vi "NPC3SG Read Data.vi"(0 "VISA resource name in":refnum<visa-resource-name>, 3 "error in":errorcluster) -> (7 "error ende":errorcluster caption="error out" {"code" format="%x"})   [LabVIEW 2010]
uses:
  drivers/Newport NPC3SG/SubNPC3SG.llb/device variables.vi
panel:
  out "Read OK":bool caption="Daten empfangen?"
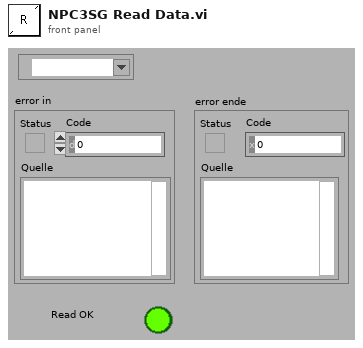
[diagram p1: front panel]
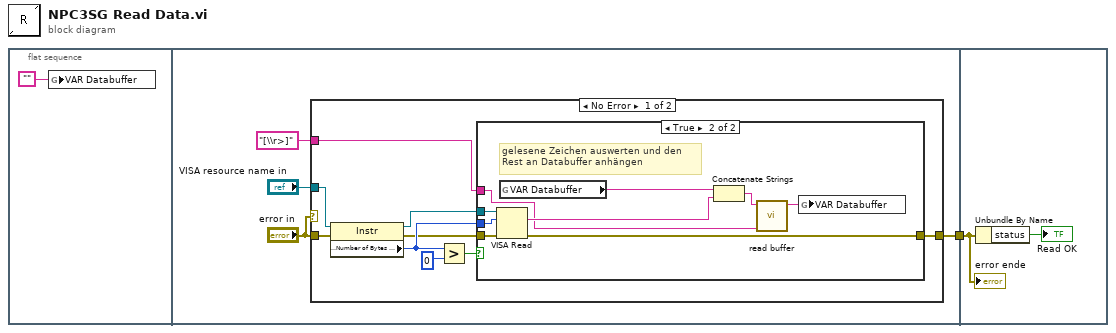
[diagram p0: block diagram]
diagram:
  n1 = flat-sequence {
    tunnel: [w5] -> w1
    tunnel: w1 -> [w27]
    frame #0 {
      n2 = global write "device variables.vi" "VAR Databuffer"("" ("VAR Databuffer")) -> ()
    }
    frame #1 {
      n3 = case shown="No Error" "error in" {
        tunnel: "[\\r>]" -> [w10 _]
        tunnel: "VISA resource name in" -> [w9 _]
        tunnel: "error in" -> [w8 w26]
        tunnel: [w7 w26] -> w5
        frame No Error {
          n4 = property class="Instr"(reference=w9, error in=w8) -> (reference out=w13:refnum<visa-resource-name>, error out=w14:errorcluster, "Serial Settings:Number of Bytes at Serial Port"=w15:u32)
          n5 = Greater?(x=w15, y=u32 0) -> (0:w12:bool)
          n6 = case shown="True" w12 {
            tunnel: w13 -> [_ w25]
            tunnel: w14 -> [w16 w24]
            tunnel: w15 -> [_ w23]
            tunnel: w10 -> [_ w18]
            tunnel: [w16 w17] -> w7
            frame False {
            }
            frame True {
              # "gelesene Zeichen auswerten und den \nRest an Databuffer anhängen"
              n7 = VISA Read(VISA resource name=w25, byte count=w23, error in (no error)=w24) -> (read buffer=w21:string, error out=w17:errorcluster)  [unwired: 2 out]
              n8 = global read "device variables.vi" "VAR Databuffer"() -> (w22:string)
              n9 = Concatenate Strings(w22, w21) -> (w20:string)
              n10 = call "read buffer.vi"("String search"=w18, "String In"=w20) -> ("String Out"=w19:string)  [unwired: 9 in]
              n11 = global write "device variables.vi" "VAR Databuffer"(w19) -> ()
            }
          }
        }
        frame Error {
        }
      }
    }
    frame #2 {
      n12 = Unbundle By Name(w27) -> ("status"=→"Read OK":bool)
      "error ende" <- w27
    }
  }
